vi "NI-DP_SearchForDevices.vi"(5 "RX Port No.":u16, 6 "timeout [ms]":u32, 7 "IP to write to":string, 8 "error in (no error)":errorcluster, 11 "UDP Network Connection in":refnum<k16>) -> (0 "error out":errorcluster, 3 "UDP Network Connection out":refnum<k16>)   [LabVIEW 2014, in "hse-network.lvlib"]
doc: "____\nHAMPEL SOFTWARE ENGINEERING v0.7.0 (2018-07-16 18:12)"
uses:
  hse-network.lvlib
  NI-DP__Commands.ctl
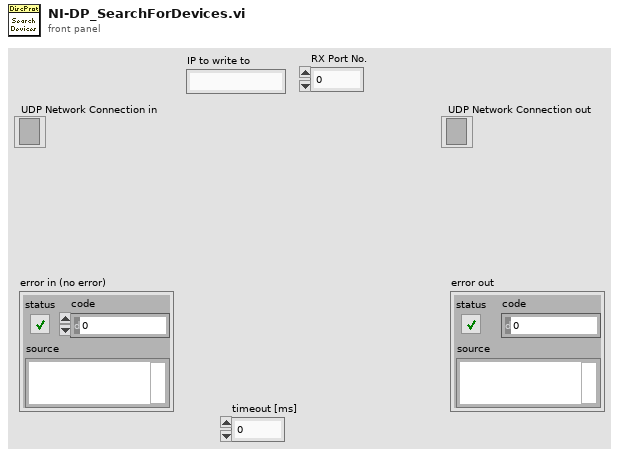
[diagram p1: front panel]
types:
  T1 = typedef "hse-network.lvlib/NI-DP__Commands.ctl" = u8
  T2 = typedef "hse-network.lvlib/NI-DP__MessageStructure.ctl" = cluster{"Start of Message":string, "Command":T1, "Checksum(?) for P3,P4":string, "Always 0x02":string, "Model Code":string, "??? 1":string, "Serial":string, "Device Mac Address":string, "??? 2":string, "Param 1":string, "Param 2":string, "Param 3":string, "Param 4":string, "Checksum(?) for Network":string, "Device IP Address":string, "Device Subnet Mask":string, "Device DNS-Server":string, "Device Default Gateway":string, "??? 3":string, "End of Message":string}
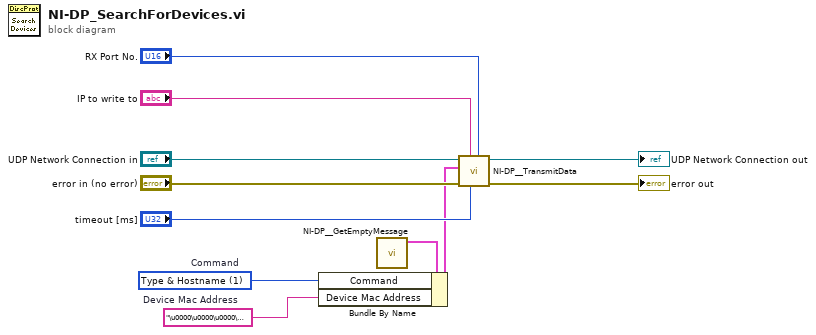
[diagram p0: block diagram]
diagram:
  w2 = "\u0000\u0000\u0000\u0000\u0000\u0000"  # Device Mac Address
  w3 = T1 1 items=["Type & Hostname"=1, "System State"=242, "Response"=32]  # Command
  n1 = call "NI-DP__GetEmptyMessage.vi"() -> ("NI-DP__EmptyMessage"=w1:T2)  [unwired: 11 in]
  n2 = Bundle By Name(cluster=w1, "Command"=w3, "Device Mac Address"=w2) -> (w4:T2)
  n3 = call "NI-DP__TransmitData.vi"("Port to write to"="RX Port No.", "timeout ms"="timeout [ms]", "IP to write to"="IP to write to", "error in"="error in (no error)", "UDP-NI__Message"=w4, "UDP Network Connection in"="UDP Network Connection in") -> ("error out"=→"error out":errorcluster, "UDP Network Connection out"=→"UDP Network Connection out":refnum<k16>)  [unwired: 4 in]
